vi "Destroy.vi"(8 "error in (no error)":errorcluster) -> (0 "error out":errorcluster)   [LabVIEW 2020, in "Configuration Manager.lvclass"]
uses:
  Configuration Manager.lvclass
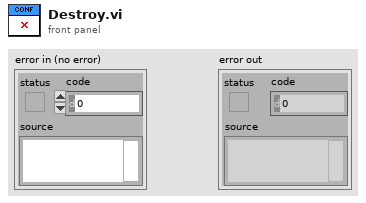
[diagram p1: front panel]
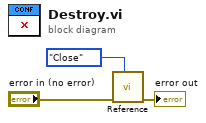
[diagram p0: block diagram]
diagram:
  n1 = call "Reference.vi"("Action"=enum16{"Get", "Close"}."Close", "error in (no error)"="error in (no error)") -> ("error out"=→"error out":errorcluster)  [unwired: 8 in, 1 out]
